vi "Move Forwards.vi"(8 "error in (no error)":errorcluster, 11 "Snake in":refnum<class "Snake.lvclass">) -> (0 "error out":errorcluster, 1 "Deleted Tail":T1, 2 "New Head":T1, 3 "Snake out":refnum<class "Snake.lvclass">)   [LabVIEW 2018, in "Snake.lvclass"]
uses:
  Snake.lvclass
  Type Defs/Coordinates.ctl
  Snake.lvclass/Snake.ctl
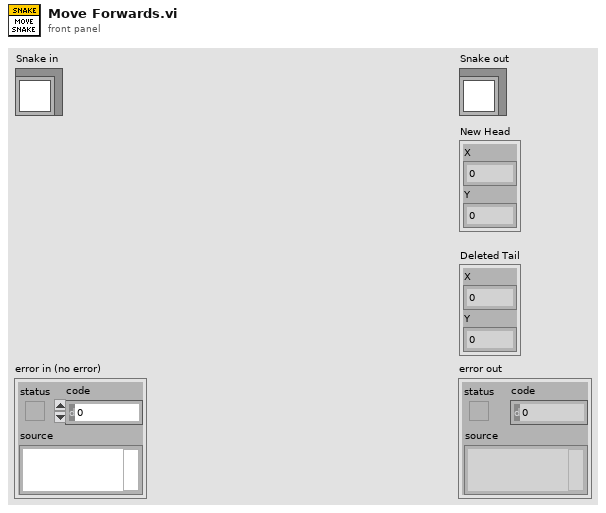
[diagram p1: front panel]
types:
  T1 = typedef "Coordinates.ctl" = cluster{"X":i32, "Y":i32}
  T2 = typedef "Direction.ctl" = enum16{"Up", "Down", "Left", "Right"}
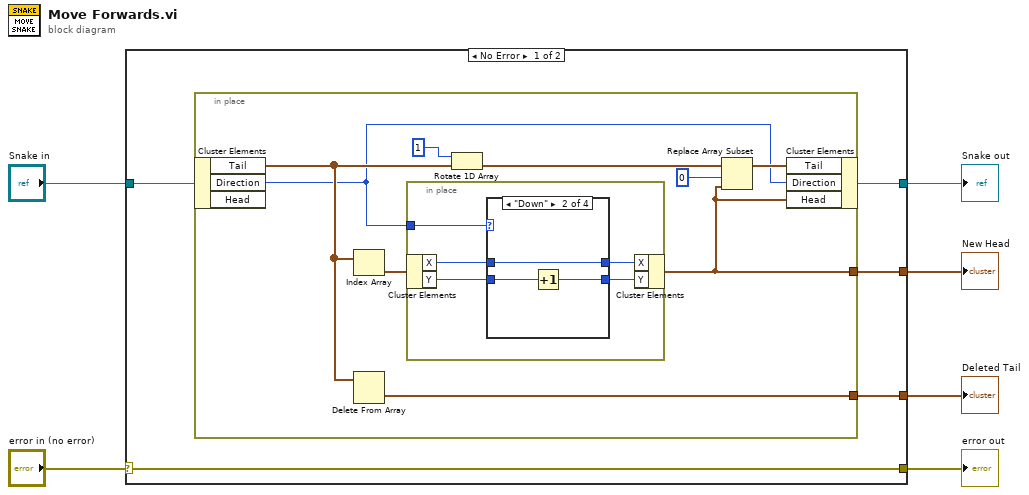
[diagram p0: block diagram]
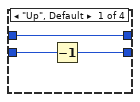
[diagram p2: hidden frame]
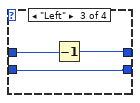
[diagram p3: hidden frame]
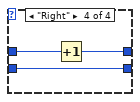
[diagram p4: hidden frame]
diagram:
  n1 = case shown="No Error" "error in (no error)" {
    selector: "error in (no error)" -> [w11 w39]
    tunnel: [w11 w39] -> w5
    tunnel: [w7 w38] -> w3
    tunnel: "Snake in" -> [w8 w38]
    tunnel: [w10 _] -> w2
    tunnel: [w9 _] -> w1
    frame No Error {
      n2 = in-place {
        in-place-border: [w18] -> w10
        in-place-border: [w12] -> w9
        n3 = in-place-cluster #1(w8) -> ("Tail"=w15:T1[], "Direction"=w13:T2)  [unwired: 1 out]
        n4 = Index Array(array=w15) -> (element=w16:T1)  [unwired: 1 in]
        n5 = Delete From Array(array=w15) -> (deleted portion=w18:T1)  [unwired: 2 in, 1 out]
        n6 = in-place {
          in-place-border: w13 -> [w25]
          n7 = in-place-cluster #2(w16) -> ("X"=w23:i32, "Y"=w24:i32)
          n8 = case shown="\"Down\"" w25 {
            tunnel: w23 -> [w27 w30 w33 w35]
            tunnel: w24 -> [w26 w29 w32 w36]
            tunnel: [w27 w30 w34 w37] -> w22
            tunnel: [w28 w31 w32 w36] -> w21
            frame "Up", Default {
              n9 = Decrement(x=w26) -> (x-1=w28:i32)
            }
            frame "Down" {
              n10 = Increment(x=w29) -> (x+1=w31:i32)
            }
            frame "Left" {
              n11 = Decrement(x=w33) -> (x-1=w34:i32)
            }
            frame "Right" {
              n12 = Increment(x=w35) -> (x+1=w37:i32)
            }
          }
          n13 = in-place-cluster #2("X"=w22, "Y"=w21) -> (w12:T1)
        }
        n14 = Rotate 1D Array(1:w15, 2:1 ("n")) -> (0:w17:T1[])
        n15 = Replace Array Subset(array=w17, new element=w12, index=0) -> (w14:T1[])
        n16 = in-place-cluster #1("Tail"=w14, "Direction"=w13, "Head"=w12) -> (w7:refnum<class "Snake.lvclass">)
      }
    }
    frame Error {
    }
  }
  "error out" <- w5
  "Snake out" <- w3
  "Deleted Tail" <- w2
  "New Head" <- w1
